vi "4 DDS 8SPC.vi"(8 "input valid":bool=TRUE, 9 "pdw in":T2 {"frequency shift" format="%#_12f"}, 10 "free DDS before me?":bool, 11 "new PDW in":bool) -> (0 "output valid":bool, 1 "state of every DDS":bool[](array[boolean]), 2 "have free DDS":bool, 3 "IQ out":T1[](array[typedef]))   [LabVIEW 2021]
doc: "transmit pulse with one free DDS inside.\nmust have no DDS before him (the distribute is to give the lowest mun DDS the pulse)"
uses:
  pulse_tx_vis/pdw.ctl
  pulse_tx_vis/mode_type.ctl
  <instrlib>/_niInstr/DSP/v1/Shared/Public/IQ Data.ctl
  <instrlib>/_niInstr/DSP/v1/Shared/niInstr DSP v1 Shared.lvlib
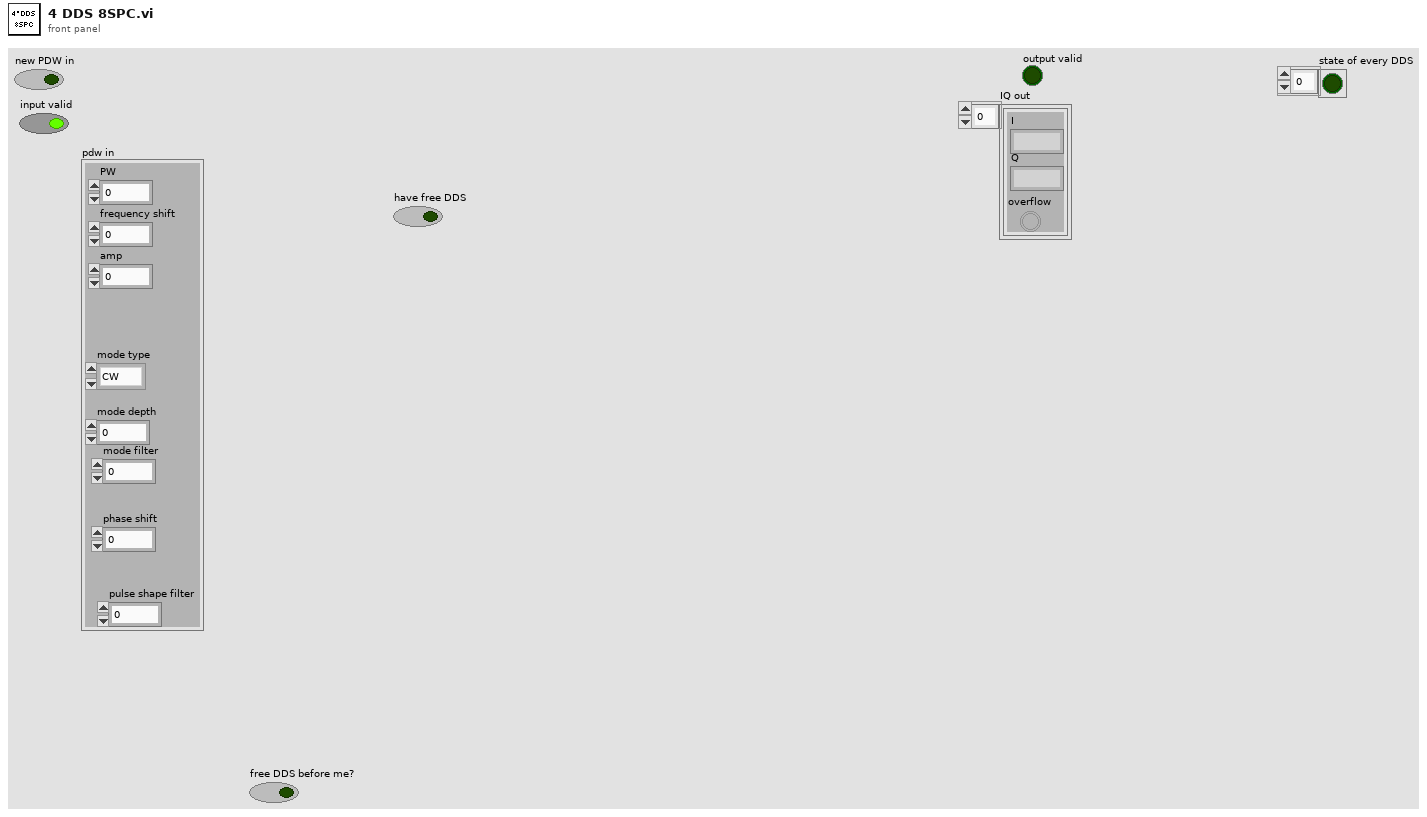
[diagram p1: front panel]
types:
  T1 = typedef "niInstr DSP v1 Shared.lvlib/IQ Data.ctl" = cluster{"I":fxp<+/-,18,1>, "Q":fxp<+/-,18,1>, "overflow":bool}
  T2 = typedef "pdw.ctl" = cluster{"PW":u32, "frequency shift":fxp<+/-,48,0>, "amp":fxp<+/-,18,1>, "mode type":T3, "mode depth":u32, "mode filter":u8, "phase shift":fxp<+/-,16,1>, "pulse shape filter":u8}
  T3 = typedef "mode_type.ctl" = enum8{"CW", "NC - CW", "NC - cw", "LFM", "BPSK", "QPSK"}
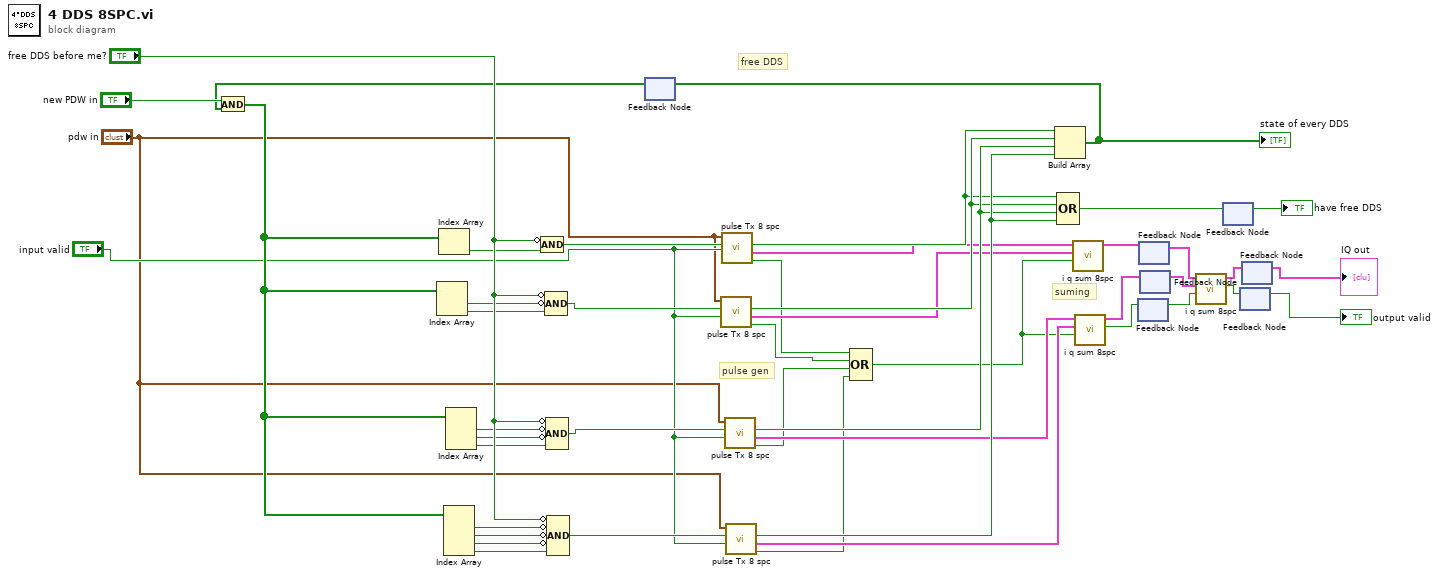
[diagram p0: block diagram]
diagram:
  # "free DDS"
  # "suming"
  # "pulse gen"
  n1 = feedback #1() -> (w21:bool[])  [unwired: 1 in]
  n2 = And(x="new PDW in", y=w21) -> (x .and. y?=w20:bool[])
  n3 = Index Array(array=w20) -> (element #1=w32:bool, element #2=w30:bool)  [unwired: 2 in]
  n4 = Index Array(array=w20) -> (element=w28:bool)  [unwired: 1 in]
  n5 = Index Array(array=w20) -> (element #1=w40:bool, element #2=w39:bool, element #3=w38:bool, element #4=w37:bool)  [unwired: 4 in]
  n6 = Index Array(array=w20) -> (element #1=w36:bool, element #2=w35:bool, element #3=w34:bool)  [unwired: 3 in]
  n7 = Compound Arithmetic op=AND(invert "free DDS before me?", w28) -> (w29:bool)
  n8 = Compound Arithmetic op=AND(invert "free DDS before me?", invert w32, w30) -> (w31:bool)
  n9 = Compound Arithmetic op=AND(invert "free DDS before me?", invert w36, invert w35, w34) -> (w33:bool)
  n10 = Compound Arithmetic op=AND(invert "free DDS before me?", invert w40, invert w39, invert w38, w37) -> (w41:bool)
  n11 = call "pulse Tx 8 spc.vi"("enable line"="input valid", "take it!"=w31, "Cluster"="pdw in") -> ("output valid"=w14:bool, "IQ out"=w25:T1[], "free dds"=w43:bool)  [unwired: 4 in, 2 out]
  n12 = call "pulse Tx 8 spc.vi"("enable line"="input valid", "take it!"=w29, "Cluster"="pdw in") -> ("output valid"=w15:bool, "IQ out"=w24:T1[], "free dds"=w42:bool)  [unwired: 4 in, 2 out]
  n13 = call "pulse Tx 8 spc.vi"("enable line"="input valid", "take it!"=w33, "Cluster"="pdw in") -> ("output valid"=w13:bool, "IQ out"=w26:T1[], "free dds"=w44:bool)  [unwired: 4 in, 2 out]
  n14 = call "pulse Tx 8 spc.vi"("enable line"="input valid", "take it!"=w41, "Cluster"="pdw in") -> ("output valid"=w12:bool, "IQ out"=w27:T1[], "free dds"=w45:bool)  [unwired: 4 in, 2 out]
  n15 = Compound Arithmetic op=OR(w15, w14, w13, w12) -> (w11:bool)
  n16 = Build Array(w42, w43, w44, w45) -> (w23:bool[])
  "state of every DDS" <- w23
  n17 = feedback-in #1(w23) -> ()
  n18 = Compound Arithmetic op=OR(w42, w43, w44, w45) -> (w19:bool)
  n19 = call "i q sum 8spc.vi"("input valid"=w11, "IQ in 2"=w25, "IQ in"=w24) -> ("IQ out"=w10:T1[])  [unwired: 7 in, 1 out]
  n20 = call "i q sum 8spc.vi"("input valid"=w11, "IQ in 2"=w27, "IQ in"=w26) -> ("output valid"=w8:bool, "IQ out"=w9:T1[])  [unwired: 7 in]
  n21 = feedback-in #2(w8) -> ()
  n22 = feedback #2() -> (w7:bool)  [unwired: 1 in]
  n23 = feedback #3() -> (w5:T1[])  [unwired: 1 in]
  n24 = feedback-in #3(w10) -> ()
  n25 = feedback #4() -> (w6:T1[])  [unwired: 1 in]
  n26 = feedback-in #4(w9) -> ()
  n27 = call "i q sum 8spc.vi"("input valid"=w7, "IQ in 2"=w6, "IQ in"=w5) -> ("output valid"=w2:bool, "IQ out"=w4:T1[])  [unwired: 7 in]
  n28 = feedback #5() -> (→"have free DDS":bool)  [unwired: 1 in]
  n29 = feedback-in #5(w19) -> ()
  n30 = feedback #6() -> (→"output valid":bool)  [unwired: 1 in]
  n31 = feedback-in #6(w2) -> ()
  n32 = feedback #7() -> (→"IQ out":T1[])  [unwired: 1 in]
  n33 = feedback-in #7(w4) -> ()
